vi "Main.vi"   [LabVIEW 2021]
uses:
  <vilib>/addons/Qbus/Qbus.lvclass
  processes/ManageConnection/AudioGenManageConnection.lvlib
  shared/logger process/EventLoggerProcess.lvlib
  <vilib>/addons/PointValueMap/PointValueMap.lvlib
  processes/TCP Read/AudioGenTCPReader.lvlib
  processes/Digital Audio Generation/DigialAudioGeneration.lvlib
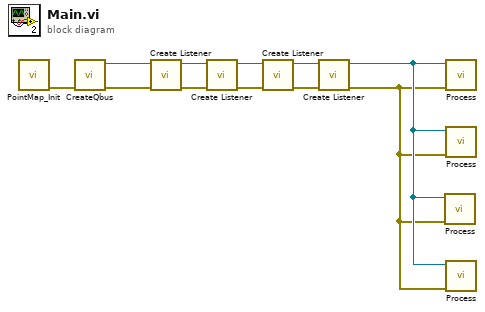
[diagram p0: block diagram]
diagram:
  n1 = call <vilib>:"PointMap_Init.vi"() -> ("error out"=w9:errorcluster)  [unwired: 11 in]
  n2 = call <vilib>:"CreateQbus.vi"("error in (no error)"=w9) -> ("error out"=w10:errorcluster, "Qbus"=w11:refnum<class "Qbus.lvclass">)  [unwired: 9 in]
  n3 = call "Create Listener.vi"("error in (no error)"=w10, "Qbus in"=w11) -> ("error out"=w8:errorcluster, "Qbus out"=w7:refnum<class "Qbus.lvclass">)  [unwired: 8 in]
  n4 = call "Create Listener.vi"("error in (no error)"=w8, "Qbus in"=w7) -> ("error out"=w5:errorcluster, "Qbus out"=w6:refnum<class "Qbus.lvclass">)  [unwired: 8 in]
  n5 = call "Create Listener.vi"("error in (no error)"=w5, "Qbus in"=w6) -> ("error out"=w3:errorcluster, "Qbus out"=w4:refnum<class "Qbus.lvclass">)  [unwired: 8 in]
  n6 = call "Create Listener.vi"("error in (no error)"=w3, "Qbus in"=w4) -> ("error out"=w1:errorcluster, "Qbus out"=w2:refnum<class "Qbus.lvclass">)  [unwired: 8 in]
  n7 = call "Process.vi"("error in"=w1, "Qbus in"=w2) -> ()  [unwired: 9 in, 1 out]
  n8 = call "Process.vi"("error in"=w1, "Qbus in"=w2) -> ()  [unwired: 9 in, 1 out]
  n9 = call "Process.vi"("error in"=w1, "Qbus in"=w2) -> ()  [unwired: 9 in, 1 out]
  n10 = call "Process.vi"("error in"=w1, "Qbus in"=w2) -> ()  [unwired: 9 in, 1 out]
